vi "Create new class icon user layers.vi"(8 "new picture":picture, 9 "LayerName":string, 10 "String in":string, 11 "RW glyph":picture) -> (3 "User Layers":refnum<class "Layer.lvclass">[](array[class]))   [LabVIEW 2021]
uses:
  vi.lib/LabVIEW Icon API/lv_icon/Classes/Layer/Layer.lvclass
  vi.lib/LabVIEW Icon API/lv_icon/Controls/Layer.ctl
  vi.lib/LabVIEW Icon API/lv_icon/lv_icon.lvlib
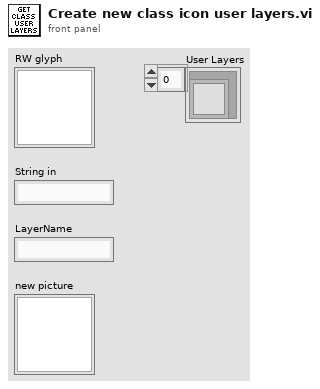
[diagram p1: front panel]
types:
  T1 = typedef "Layer.ctl" = cluster{"LayerIcon":picture, "LayerName":string, "Opacity":u8, "Visibility?":bool}
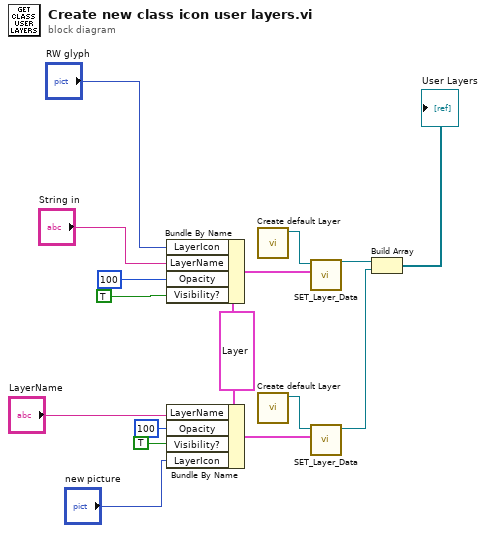
[diagram p0: block diagram]
diagram:
  w8 = T1 {"LayerIcon"=bytes[3102], "LayerName"="", "Opacity"=100, "Visibility?"=TRUE} ("Data")
  n1 = Bundle By Name(cluster=w8, "LayerIcon"="RW glyph", "LayerName"="String in", "Opacity"=u8 100, "Visibility?"=TRUE) -> (w6:T1)
  n2 = Bundle By Name(cluster=w8, "LayerName"="LayerName", "Opacity"=u8 100, "Visibility?"=TRUE, "LayerIcon"="new picture") -> (w9:T1)
  n3 = call "Create default Layer.vi"() -> ("Layer.lvclass out"=w1:refnum<class "Layer.lvclass">)  [unwired: 1 in, 10 out]
  n4 = call "Create default Layer.vi"() -> ("Layer.lvclass out"=w7:refnum<class "Layer.lvclass">)  [unwired: 1 in, 10 out]
  n5 = call-dynamic "SET_Layer_Data.vi"("Data"=w6, "Layer.lvclass in"=w1) -> ("Layer.lvclass out"=w14:refnum<class "Layer.lvclass">)  [unwired: 2 in, 7 out]
  n6 = call-dynamic "SET_Layer_Data.vi"("Data"=w9, "Layer.lvclass in"=w7) -> ("Layer.lvclass out"=w15:refnum<class "Layer.lvclass">)  [unwired: 2 in, 7 out]
  n7 = Build Array(w14, w15) -> (→"User Layers":refnum<class "Layer.lvclass">[])
